vi "WriteIO.loop.fpga.vi"(9 "Delta time":u32, 10 "Number of time points":i32) -> ()   [LabVIEW 2012]
uses:
  <vilib>/Platform/TimedLoop/XDataNode/timing_clust.ctl
  <vilib>/Platform/TimedLoop/XDataNode/nitl_modes.ctl
  <vilib>/Platform/TimedLoop/XDataNode/wakeup.ctl
  <vilib>/rvi/interface/RandomDataEmulation/nirviRandomDataFPGAFIFO.vi
  <vilib>/rvi/interface/RandomDataEmulation/niFpgaRandomDataHandleErrors.vi
  <vilib>/rvi/Emulation/niFpgaSctlEmulationRegisterWithScheduler.vi
  <vilib>/rvi/Emulation/niFpgaSctlEmulationScheduler.vi
  <vilib>/rvi/eio/common/nirviEmuTemplateMethod_errors.vi
  <vilib>/platform/TimedLoop/XDataNode/XDataNode.xnode
  <vilib>/rvi/DataTransferAndStorage/Container/XNode/niFpgaContainer.xnode
  <vilib>/rvi/interface/RandomDataEmulation/nirviRandomDataFpgaReadWriteTemplate.vi
  <vilib>/eio/EIONode/EIONode.xnode
  <vilib>/Platform/TimedLoop/XDataNode/XDNodeRunTimeDep.lvlib
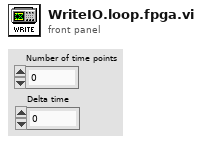
[diagram p1: front panel]
types:
  T1 = typedef "XDNodeRunTimeDep.lvlib/timing_clust.ctl" = cluster{"Expected End [f-1]":u64, "Actual End [f-1]":u64, "Finished Late? [f-1]":bool, "Expected End [i-1]":u64, "Actual End [i-1]":u64, "Finished Late? [i-1]":bool, "Expected Start [i]":u64, "Actual Start [i]":u64, "Expected Start [f]":u64, "Actual Start [f]":u64, "Source Name":string, "Structure Name":string, "Period":i64, "Deadline":i64, "Offset":i64, "Start":i64, "Priority":i32, "Timeout":i32, "Mode":T2, "Wakeup Reason":T3, "Error":errorcluster, "Source Type":string, "Secondary Source Type":string, "Global End Time":u64, "Global Start Time":u64, "Frame Duration":u64, "Iteration Duration":u64, "Assigned CPU":i32, "I/O Scan Engine Mode":u32}
  T2 = typedef "XDNodeRunTimeDep.lvlib/nitl_modes.ctl" = enum32{"No Change", "Process missed periods, maintain original phase", "Discard missed periods, maintain original phase", "Process missed periods, ignore original phase", "Discard missed periods, ignore original phase"}
  T3 = typedef "XDNodeRunTimeDep.lvlib/wakeup.ctl" = enum32{"Normal", "Aborted", "Asynchronous wakeup", "Timing source error", "Timed loop error", "Timeout"}
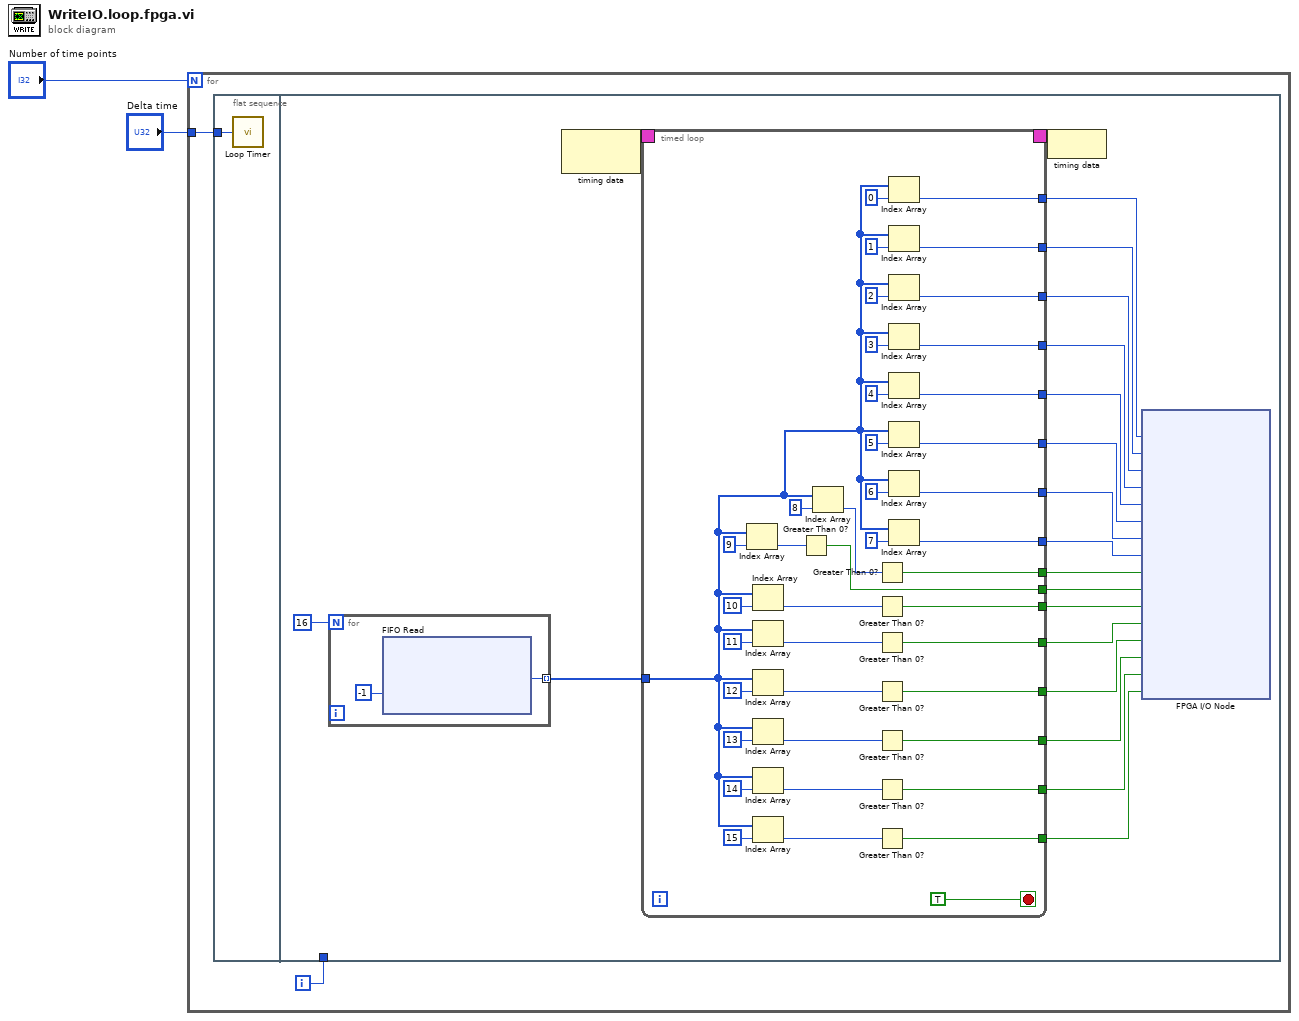
[diagram p0: block diagram]
diagram:
  n1 = for {
    N: "Number of time points" -> [_]
    tunnel: "Delta time" -> [w4]
    i -> [w3]
    n2 = flat-sequence {
      tunnel: w4 -> [w5]
      tunnel: w3 -> [_]
      frame #0 {
        n3 = call "Loop Timer"("Count(Ticks)"=w5) -> ()  [unwired: 1 out]
      }
      frame #1 {
        n4 = for {
          N: 16 -> [_]
          tunnel: [w73] -> w24 mode=indexing
          n5 = xnode "FIFO Read"("Timeout"=-1) -> ("Element"=w73:i16)  [unwired: 1 in, 2 out]
        }
        n6 = node-c288() -> (w22:T1)  [unwired: 1 in]
        n7 = timed-loop {
          timing: w22 -> [_]
          timing-out: [_] -> w21
          tunnel: w24 -> [w49]
          tunnel: [w67] -> w23
          tunnel: [w64] -> w20
          tunnel: [w48] -> w19
          tunnel: [w47] -> w18
          tunnel: [w46] -> w17
          tunnel: [w45] -> w16
          tunnel: [w44] -> w15
          tunnel: [w43] -> w14
          tunnel: [w42] -> w13
          tunnel: [w39] -> w12
          tunnel: [w37] -> w11
          tunnel: [w35] -> w10
          tunnel: [w33] -> w9
          tunnel: [w31] -> w8
          tunnel: [w29] -> w7
          tunnel: [w27] -> w6
          stop <- TRUE stop-if-true
          n8 = Index Array(array=w49, index=9) -> (element=w40:i16)
          n9 = Index Array(array=w49, index=10) -> (element=w38:i16)
          n10 = Index Array(array=w49, index=11) -> (element=w36:i16)
          n11 = Index Array(array=w49, index=12) -> (element=w34:i16)
          n12 = Index Array(array=w49, index=13) -> (element=w32:i16)
          n13 = Index Array(array=w49, index=14) -> (element=w30:i16)
          n14 = Index Array(array=w49, index=15) -> (element=w28:i16)
          n15 = Greater Than 0?(x=w40) -> (x > 0?=w39:bool)
          n16 = Index Array(array=w49, index=8) -> (element=w41:i16)
          n17 = Greater Than 0?(x=w41) -> (x > 0?=w42:bool)
          n18 = Greater Than 0?(x=w38) -> (x > 0?=w37:bool)
          n19 = Greater Than 0?(x=w36) -> (x > 0?=w35:bool)
          n20 = Greater Than 0?(x=w34) -> (x > 0?=w33:bool)
          n21 = Greater Than 0?(x=w32) -> (x > 0?=w31:bool)
          n22 = Greater Than 0?(x=w30) -> (x > 0?=w29:bool)
          n23 = Greater Than 0?(x=w28) -> (x > 0?=w27:bool)
          n24 = Index Array(array=w49, index=0) -> (element=w67:i16)
          n25 = Index Array(array=w49, index=1) -> (element=w64:i16)
          n26 = Index Array(array=w49, index=2) -> (element=w48:i16)
          n27 = Index Array(array=w49, index=3) -> (element=w47:i16)
          n28 = Index Array(array=w49, index=4) -> (element=w46:i16)
          n29 = Index Array(array=w49, index=5) -> (element=w45:i16)
          n30 = Index Array(array=w49, index=6) -> (element=w44:i16)
          n31 = Index Array(array=w49, index=7) -> (element=w43:i16)
        }
        n32 = node-c288(w21) -> ()
        n33 = xnode "FPGA I/O Node"("Connector0/AO0"=w23, "Connector0/AO1"=w20, "Connector0/AO2"=w19, "Connector0/AO3"=w18, "Connector0/AO4"=w17, "Connector0/AO5"=w16, "Connector0/AO6"=w15, "Connector0/AO7"=w14, "Connector0/DIO0"=w13, "Connector0/DIO1"=w12, "Connector0/DIO2"=w11, "Connector0/DIO3"=w10, "Connector0/DIO4"=w9, "Connector0/DIO5"=w8, "Connector0/DIO6"=w7, "Connector0/DIO7"=w6) -> ()  [unwired: 16 in, 16 out]
      }
    }
  }
